vi "write current Lens Driver.vi"(0 "VISA resource name":refnum<visa-resource-name>, 1 "Max Current A":dbl, 2 "Max Current B":dbl, 5 "Current":T5={"Current dc A"=0.0, "Current dc B"=0.0, "Frequency A"=0.0, "Frequency B"=0.0, "Current hi A"=0.0, "Current hi B"=0.0, "Current low A"=0.0, "Current low B"=0.0, "Focal Power A"=3.0, "Temperature high A"=20.0, "Temperature low A"=45.0} {"Current dc A" scale=-200.0..200.0 scale format="%#_5g"; "Current dc B" scale=-200.0..200.0 scale format="%#_5g"; "Frequency A" scale=0.1..1000.0; "Frequency B" scale=0.1..1000.0; "Current hi A" scale=-200.0..200.0 scale format="%#_5g"; "Current hi B" scale=-200.0..200.0 scale format="%#_5g"; "Current low A" scale=-200.0..200.0 scale format="%#_5g"; "Current low B" scale=-200.0..200.0 scale format="%#_5g"; "Focal Power A" scale=-5.0..10.0 scale format="%#_5g"; "Temperature high A" scale=10.0..100.0; "Temperature low A" scale=10.0..100.0}, 11 "error in (no error)":errorcluster) -> (3 "Current 3":T5={"Current dc A"=0.0, "Current dc B"=0.0, "Frequency A"=0.0, "Frequency B"=0.0, "Current hi A"=0.0, "Current hi B"=0.0, "Current low A"=0.0, "Current low B"=0.0, "Focal Power A"=3.0, "Temperature high A"=20.0, "Temperature low A"=45.0} {"Current dc A" scale=-200.0..200.0 scale format="%#_5g"; "Current dc B" scale=-200.0..200.0 scale format="%#_5g"; "Frequency A" scale=0.1..1000.0; "Frequency B" scale=0.1..1000.0; "Current hi A" scale=-200.0..200.0 scale format="%#_5g"; "Current hi B" scale=-200.0..200.0 scale format="%#_5g"; "Current low A" scale=-200.0..200.0 scale format="%#_5g"; "Current low B" scale=-200.0..200.0 scale format="%#_5g"; "Focal Power A" scale=-5.0..10.0 scale format="%#_5g"; "Temperature high A" scale=10.0..100.0; "Temperature low A" scale=10.0..100.0}, 4 "VISA resource name out":refnum<visa-resource-name>, 8 "OK":bool, 15 "error out":errorcluster)   [LabVIEW 2013]
doc: "This VI allows a fast changing of current values over global variables (Global Lens Driver.vi) which can be feed by a parallel running VI. Runs continously if global variable \"Run\" is true."
uses:
  03 Type Def & Global/Slider.ctl
  03 Type Def & Global/Slider Freq.ctl
  03 Type Def & Global/Slider Focal Power.ctl
  03 Type Def & Global/Slider Temperature.ctl
  03 Type Def & Global/Global Lens Driver.vi
panel:
  in  "Stop Button":bool
  in  "Current dc B":dbl(slide) scale=0.1..1000.0
  in  "Current dc A":dbl(slide) scale=0.1..1000.0
  out "x-y":u32
  out "write":string
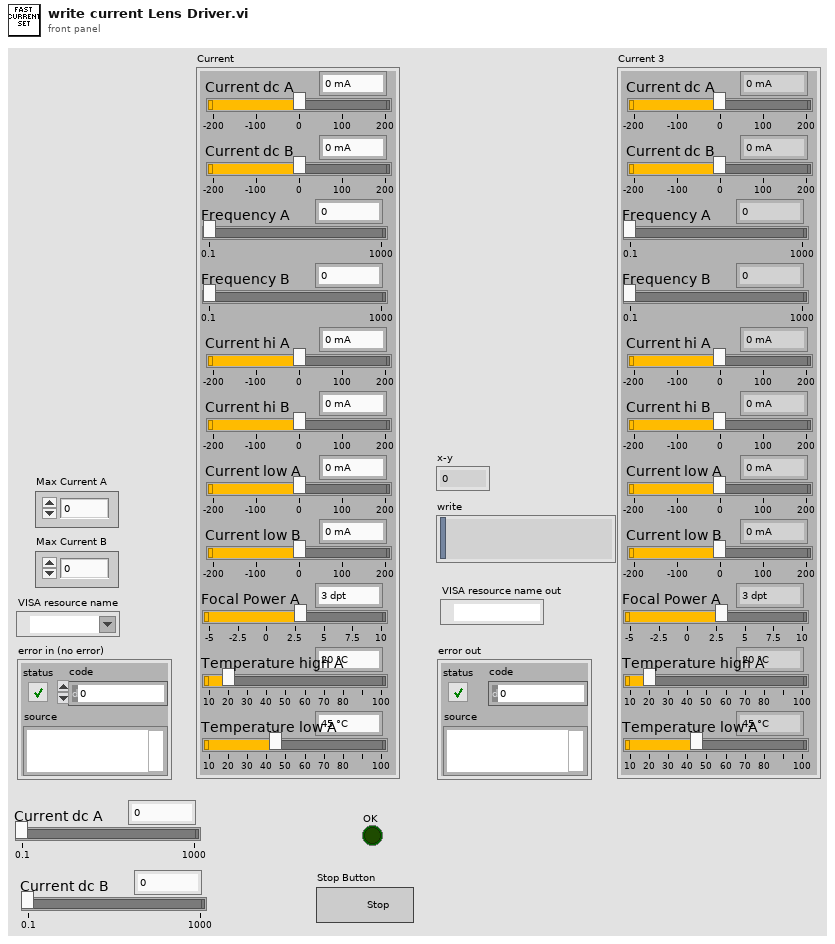
[diagram p1: front panel]
types:
  T1 = typedef "Slider.ctl" = dbl
  T2 = typedef "Slider Freq.ctl" = dbl
  T3 = typedef "Slider Focal Power.ctl" = dbl
  T4 = typedef "Slider Temperature.ctl" = dbl
  T5 = cluster{"Current dc A":T1, "Current dc B":T1, "Frequency A":T2, "Frequency B":T2, "Current hi A":T1, "Current hi B":T1, "Current low A":T1, "Current low B":T1, "Focal Power A":T3, "Temperature high A":T4, "Temperature low A":T4}
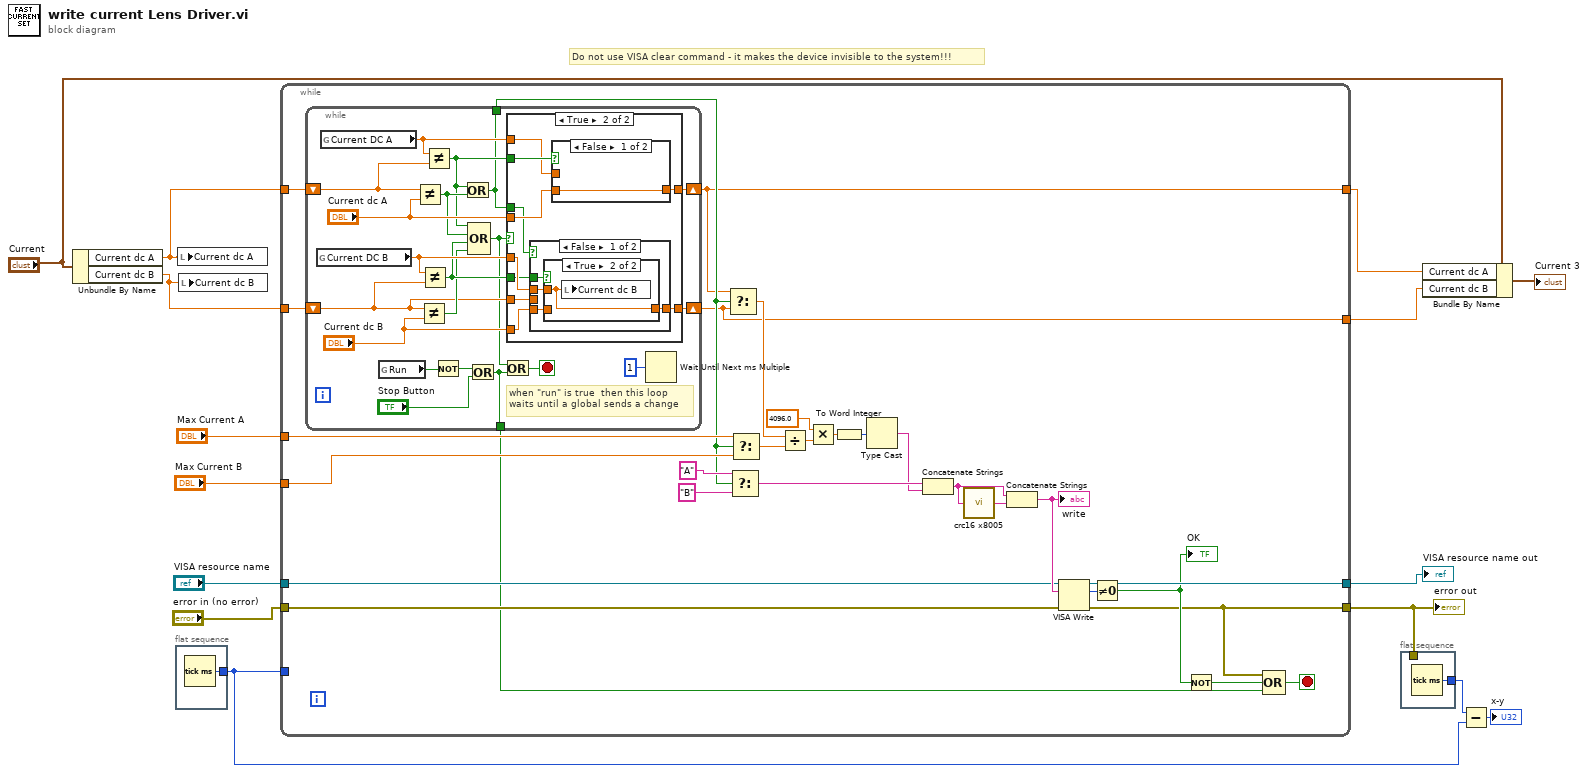
[diagram p0: block diagram]
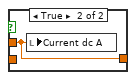
[diagram p5: hidden frame]
diagram:
  # "Do not use VISA clear command - it makes the device invisible to the system!!!"
  n1 = Unbundle By Name("Current") -> ("Current dc A"=w4:T1, "Current dc B"=w3:T1)
  n2 = flat-sequence {
    tunnel: [w16] -> _
    tunnel: [w16] -> w13
    frame #0 {
      n3 = Tick Count (ms)() -> (millisecond timer value=w16:u32)
    }
  }
  n4 = local write "Current dc A"(w4) -> ()
  n5 = local write "Current dc B"(w3) -> ()
  n6 = while {
    tunnel: w13 -> [_]
    tunnel: [w22] -> w12
    tunnel: [w42] -> w11
    tunnel: "VISA resource name" -> [w41]
    tunnel: "error in (no error)" -> [w40]
    tunnel: "Max Current A" -> [w35]
    tunnel: "Max Current B" -> [w36]
    tunnel: [w25] -> w6
    tunnel: [w24] -> w5
    tunnel: w4 -> [w21]
    tunnel: w3 -> [w20]
    stop <- w28 stop-if-true
    n7 = while {
      shift-right: [w62] -> w25
      shift-left: w21 -> [w65]
      shift-right: [w61] -> w24
      shift-left: w20 -> [w53]
      tunnel: [w54] -> w29
      tunnel: [w46] -> w26
      stop <- w51 stop-if-true
      # "when \"run\" is true  then this loop\nwaits until a global sends a change"
      n8 = global read "Global Lens Driver.vi" "Current DC B"() -> (w60:dbl)
      n9 = global read "Global Lens Driver.vi" "Current DC A"() -> (w63:dbl)
      n10 = global read "Global Lens Driver.vi" "Run"() -> (w49:bool)
      n11 = Not Equal?(x=w65, y="Current dc A") -> (x != y?=w56:bool)
      n12 = Not Equal?(x=w53, y="Current dc B") -> (x != y?=w57:bool)
      n13 = Not Equal?(x=w60, y=w53) -> (x != y?=w58:bool)
      n14 = Not Equal?(x=w63, y=w65) -> (x != y?=w55:bool)
      n15 = Not(x=w49) -> (.not. x?=w47:bool)
      n16 = Or(x=w55, y=w56) -> (x .or. y?=w54:bool)
      n17 = Compound Arithmetic op=OR(w55, w56, w58, w57) -> (w50:bool)
      n18 = Or(x=w47, y="Stop Button") -> (x .or. y?=w46:bool)
      n19 = Or(x=w50, y=w46) -> (x .or. y?=w51:bool)
      n20 = case shown="True" w50 {
        tunnel: "Current dc A" -> [w67 w75]
        tunnel: w63 -> [_ w76]
        tunnel: w55 -> [_ w77]
        tunnel: [w67 w74] -> w62
        tunnel: "Current dc B" -> [w66 w72]
        tunnel: w60 -> [_ w71]
        tunnel: w58 -> [_ w70]
        tunnel: [w66 w73] -> w61
        tunnel: w54 -> [_ w69]
        tunnel: w53 -> [_ w68]
        frame False {
        }
        frame True {
          n21 = case shown="False" w69 {
            tunnel: [w81 w84] -> w73
            tunnel: w72 -> [w80 _]
            tunnel: w71 -> [w79 _]
            tunnel: w70 -> [w78 _]
            tunnel: w68 -> [_ w84]
            frame False {
              n22 = case shown="True" w78 {
                tunnel: w79 -> [_ w83]
                tunnel: w80 -> [w82 _]
                tunnel: [w82 w83] -> w81
                frame False {
                }
                frame True {
                  n23 = local write "Current dc B"(w83) -> ()
                }
              }
            }
            frame True {
            }
          }
          n24 = case shown="False" w77 {
            tunnel: w76 -> [_ w86]
            tunnel: w75 -> [w85 _]
            tunnel: [w85 w86] -> w74
            frame False {
            }
            frame True {
              n25 = local write "Current dc A"(w86) -> ()
            }
          }
        }
      }
      n26 = Wait Until Next ms Multiple(millisecond multiple=u32 1) -> ()  [unwired: 1 out]
    }
    n27 = Select(t=w25, s=w29, f=w24) -> (s? t:f=w30:T1)
    n28 = Select(t="A" ("string (\"\")"), s=w29, f="B" ("string (\"\")")) -> (s? t:f=w31:string)
    n29 = Select(t=w35, s=w29, f=w36) -> (s? t:f=w34:dbl)
    n30 = Divide(x=w30, y=w34) -> (x/y=w38:T1)
    n31 = Multiply(x=4096.0, y=w38) -> (x*y=w18:T1)
    n32 = To Word Integer(number=w18) -> (16bit integer=w19:i16)
    n33 = Type Cast(x=w19) -> (*(type *) &x=w17:string)  [unwired: 1 in]
    n34 = Concatenate Strings(w31, w17) -> (w37:string)
    n35 = call "crc16 x8005.vi"("message"=w37) -> ("CRC16"=w45:string)  [unwired: 4 in]
    n36 = Concatenate Strings(w37, w45) -> (w44:string)
    "write" <- w44
    n37 = VISA Write(VISA resource name=w41, write buffer=w44, error in (no error)=w40) -> (VISA resource name out=w42:refnum<visa-resource-name>, return count=w43:u32, error out=w22:errorcluster)
    n38 = Not Equal To 0?(x=w43) -> (x != 0?=w27:bool)
    "OK" <- w27
    n39 = Not(x=w27) -> (.not. x?=w23:bool)
    n40 = Compound Arithmetic op=OR(w22, w23, w26) -> (w28:bool)
  }
  "error out" <- w12
  "VISA resource name out" <- w11
  n41 = flat-sequence {
    tunnel: [w87] -> w14
    tunnel: w12 -> [_]
    frame #0 {
      n42 = Tick Count (ms)() -> (millisecond timer value=w87:u32)
    }
  }
  n43 = Bundle By Name(cluster="Current", "Current dc A"=w6, "Current dc B"=w5) -> (→"Current 3":T5)
  n44 = Subtract(x=w14, y=w13) -> (x-y=→"x-y":u32)
